vi "karmienie.vi"() -> ()   [LabVIEW 2018]
panel:
  out "Czwartek":i8[](array[numeric])
  out "Środa":i8[](array[numeric])
  out "Sobota":i8[](array[numeric])
  out "Niedziela":i8[](array[numeric])
  out "Piątek":i8[](array[numeric])
  out "Wtorek":i8[](array[numeric])
  out "Poniedziałek":i8[](array[numeric])
  in  "Enum":T1(ring)
  in  "Karmienie tabela":i8[](array[numeric])=[0, 0, 0, 0, 0, 0, 0, 0, 0, 1, 0, 0, 0, 0, 0, 0, 0, 0, 2, 0, 0, 0, 0, 0, 0, 0, 0, 0, 0, 0, 0, 0, 0, 1, 0, 0, 0, 0, 0, 0, 0, 0, 2, 0, 0, 0, 0, 0, 0, 0, 0, 0, 0, 0, 0, 0, 0, 1, 0, 0, 0, 0, 0, 0, 0, 0, 2, 0, 0, 0, 0, 0, 0, 0, 0, 0, 0, 0, 0, 0, 0, 1, 0, 0, 0, 0, 0, 0, 0, 0, 2, 0, 0, 0, 0, 0, 0, 0, 0, 0, 0, 0, 0, 0, 0, 1, 0, 0, 0, 0, 0, 0, 0, 0, 2, 0, 0, 0, 0, 0, 0, 0, 0, 0, 0, 0, 0, 0, 0, 1, 0, 0, 0, 0, 0, 0, 0, 0, 2, 0, 0, 0, 0, 0, 0, 0, 0, 0, 0, 0, 0, 0, 0, 1, 0, 0, 0, 0, 0, 0, 0, 0, 2, 0, 0, 0, 0, 0]
  in  "stop":bool
  # "0 - brak pokarmu\n1 - pokarm pierwszy\n2 - pokarm drugi"
  # "Godzina"
  # "00:00"
  # "01:00"
  # "02:00"
  # "03:00"
  # "04:00"
  # "05:00"
  # "06:00"
  # "07:00"
  # "08:00"
  # "09:00"
  # "10:00"
  # "11:00"
  # "12:00"
  # "13:00"
  # "14:00"
  # "15:00"
  # "16:00"
  # "17:00"
  # "18:00"
  # "19:00"
  # "20:00"
  # "21:00"
  # "22:00"
  # "23:00"
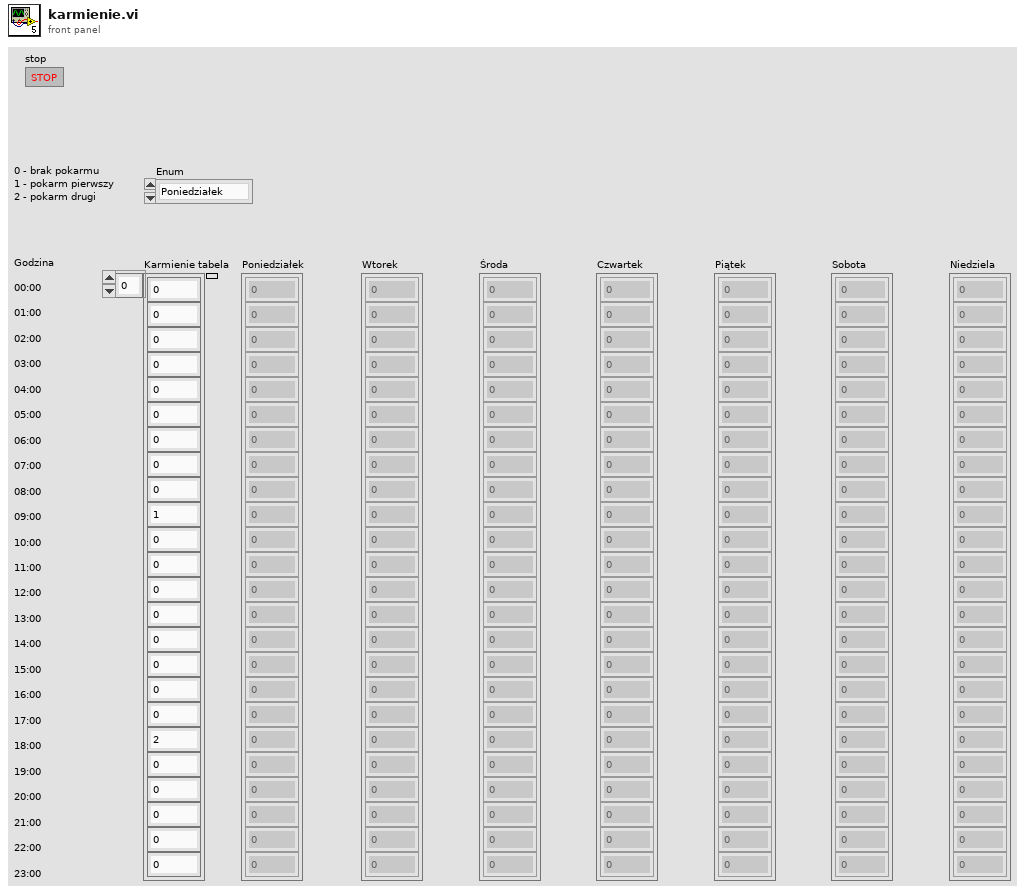
[diagram p1: front panel]
types:
  T1 = enum16{"Poniedziałek", "Wtorek", "Środa", "Czwartek", "Piątek", "Sobota", "Niedziela"}
  T2 = enum16{"big-endian, network order", "native, host order", "little-endian"}
  T3 = enum16{"open", "replace", "create", "open or create", "replace or create", "replace or create with confirmation"}
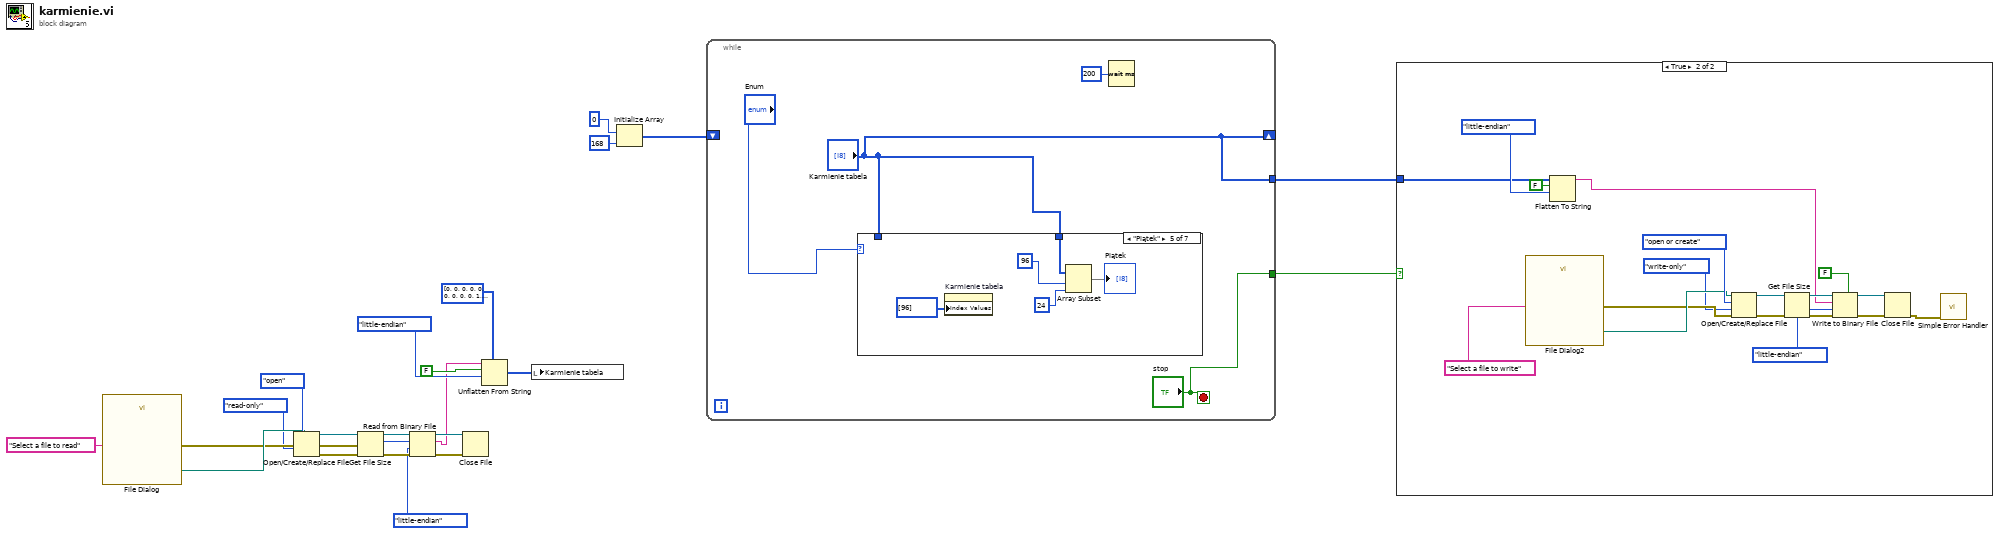
[diagram p0: block diagram]
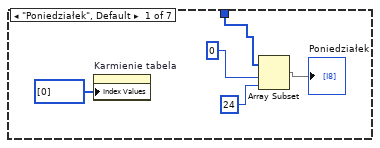
[diagram p3: hidden frame]
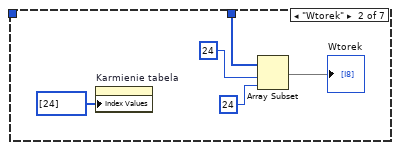
[diagram p4: hidden frame]
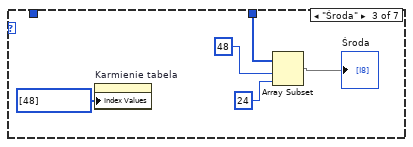
[diagram p5: hidden frame]
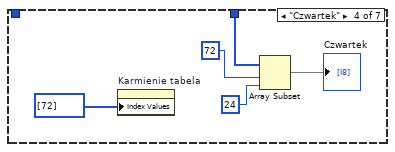
[diagram p6: hidden frame]
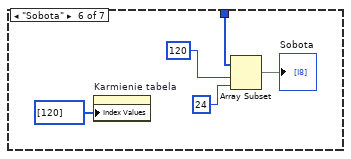
[diagram p7: hidden frame]
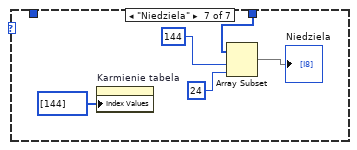
[diagram p8: hidden frame]
diagram:
  n1 = call "File Dialog"("prompt"="Select a file to read") -> ("selected path"=w11:path, "error out"=w10:errorcluster)  [unwired: 11 in, 2 out]
  n2 = Open/Create/Replace File(file path (use dialog)=w11, error in=w10, operation (0:open)=T3."open", access (0:read/write)=enum16{"read/write", "read-only", "write-only"}."read-only") -> (refnum out=w17:refnum<file>, error out=w18:errorcluster)  [unwired: 2 in, 1 out]
  n3 = Get File Size(file=w17, error in=w18) -> (refnum out=w15:refnum<file>, size (in bytes)=w4:i64, 0:w16:errorcluster)
  n4 = Read from Binary File(8:w16, 9:T2."little-endian" ("byte order (0:big-endian, network order)"), 10:w4, 11:w15) -> (0:w13:errorcluster, 2:w3:string, 3:w14:refnum<file>)  [unwired: 2 in, 1 out]
  n5 = Close File(refnum=w14, error in=w13) -> ()  [unwired: 2 out]
  n6 = Unflatten From String(type=i8[] [0, 0, 0, 0, 0, 0, 0, 0, 0, 1, 0, 0, 0, 0, 0, 0, 0, 0, 2, 0, 0, 0, 0, 0, 0, 0, 0, 0, 0, 0, 0, 0, 0, 1, 0, 0, 0, 0, 0, 0, 0, 0, 2, 0, 0, 0, 0, 0, 0, 0, 0, 0, 0, 0, 0, 0, 0, 1, 0, 0, 0, 0, 0, 0, 0, 0, 2, 0, 0, 0, 0, 0, 0, 0, 0, 0, 0, 0, 0, 0, 0, 1, 0, 0, 0, 0, 0, 0, 0, 0, 2, 0, 0, 0, 0, 0, 0, 0, 0, 0, 0, 0, 0, 0, 0, 1, 0, 0, 0, 0, 0, 0, 0, 0, 2, 0, 0, 0, 0, 0, 0, 0, 0, 0, 0, 0, 0, 0, 0, 1, 0, 0, 0, 0, 0, 0, 0, 0, 2, 0, 0, 0, 0, 0, 0, 0, 0, 0, 0, 0, 0, 0, 0, 1, 0, 0, 0, 0, 0, 0, 0, 0, 2, 0, 0, 0, 0, 0] ("Edycja"), binary string=w3, data includes array or string size? (T)=FALSE, byte order (0:big-endian, network order)=T2."little-endian") -> (value=w1:i8[])  [unwired: 1 in, 2 out]
  n7 = local write "Karmienie tabela"(w1) -> ()
  n8 = Initialize Array(i8 0 ("element"), 168 ("dimension size")) -> (w21:i8[])
  n9 = while {
    shift-right: ["Karmienie tabela"] -> _
    shift-left: w21 -> [_]
    tunnel: ["stop"] -> w20
    tunnel: ["Karmienie tabela"] -> w19
    stop <- "stop" stop-if-true
    n10 = case shown="\"Piątek\"" "Enum" {
      tunnel: "Karmienie tabela" -> [_ _ _ _ _ _ _]
      tunnel: "Karmienie tabela" -> [w30 w35 w39 w46 w50 w55 w60]
      frame "Poniedziałek", Default {
        n11 = property on="Karmienie tabela" class="Arr (strict)"("Index Values"=u32[] [0]) -> ()  [unwired: 2 in, 2 out]
        n12 = Array Subset(array=w30, index=0, length=24 ("index")) -> (→"Poniedziałek":i8[])
      }
      frame "Wtorek" {
        n13 = property on="Karmienie tabela" class="Arr (strict)"("Index Values"=u32[] [24]) -> ()  [unwired: 2 in, 2 out]
        n14 = Array Subset(array=w35, index=24, length=24 ("index")) -> (→"Wtorek":i8[])
      }
      frame "Środa" {
        n15 = property on="Karmienie tabela" class="Arr (strict)"("Index Values"=u32[] [48]) -> ()  [unwired: 2 in, 2 out]
        n16 = Array Subset(array=w39, index=48, length=24 ("index")) -> (→"Środa":i8[])
      }
      frame "Czwartek" {
        n17 = property on="Karmienie tabela" class="Arr (strict)"("Index Values"=u32[] [72]) -> ()  [unwired: 2 in, 2 out]
        n18 = Array Subset(array=w46, index=72, length=24 ("index")) -> (→"Czwartek":i8[])
      }
      frame "Piątek" {
        n19 = property on="Karmienie tabela" class="Arr (strict)"("Index Values"=u32[] [96]) -> ()  [unwired: 2 in, 2 out]
        n20 = Array Subset(array=w50, index=96, length=24 ("index")) -> (→"Piątek":i8[])
      }
      frame "Sobota" {
        n21 = property on="Karmienie tabela" class="Arr (strict)"("Index Values"=u32[] [120]) -> ()  [unwired: 2 in, 2 out]
        n22 = Array Subset(array=w55, index=120, length=24 ("index")) -> (→"Sobota":i8[])
      }
      frame "Niedziela" {
        n23 = property on="Karmienie tabela" class="Arr (strict)"("Index Values"=u32[] [144]) -> ()  [unwired: 2 in, 2 out]
        n24 = Array Subset(array=w60, index=144, length=24 ("index")) -> (→"Niedziela":i8[])
      }
    }
    n25 = Wait (ms)(milliseconds to wait=u32 200) -> ()  [unwired: 1 out]
  }
  n26 = case shown="True" w20 {
    tunnel: w19 -> [_ w63]
    frame False {
    }
    frame True {
      n27 = call "File Dialog2"("prompt"="Select a file to write") -> ("selected path"=w72:path, "error out"=w71:errorcluster)  [unwired: 11 in, 2 out]
      n28 = Flatten To String(anything=w63, prepend array or string size? (T)=FALSE, byte order (0:big-endian, network order)=T2."little-endian") -> (data string=w66:string)  [unwired: 1 in, 2 out]
      n29 = Open/Create/Replace File(file path (use dialog)=w72, error in=w71, operation (0:open)=T3."open or create", access (0:read/write)=enum16{"read/write", "read-only", "write-only"}."write-only") -> (refnum out=w79:refnum<file>, error out=w80:errorcluster)  [unwired: 2 in, 1 out]
      n30 = Get File Size(file=w79, error in=w80) -> (refnum out=w77:refnum<file>, 0:w78:errorcluster)  [unwired: 1 out]
      n31 = Write to Binary File(file (use dialog)=w77, data=w66, error in=w78, 5:FALSE ("prepend array or string size? (T)"), 9:T2."little-endian" ("byte order (0:big-endian, network order)")) -> (refnum out=w76:refnum<file>, error out=w75:errorcluster)  [unwired: 1 in, 1 out]
      n32 = Close File(refnum=w76, error in=w75) -> (error out=w69:errorcluster)  [unwired: 1 out]
      n33 = call <vilib>:"Simple Error Handler.vi"("error in (no error)"=w69) -> ()  [unwired: 4 in, 5 out]
    }
  }
